vi "Add Element.vi"(8 "Error In":errorcluster, 10 "New Element":refnum<class "Display Element.lvclass">, 11 "Display Manager In":refnum<class "Display Manager.lvclass">) -> (0 "Error Out":errorcluster, 3 "Display Manager Out":refnum<class "Display Manager.lvclass">)   [LabVIEW 2021, in "Display Manager.lvclass"]
uses:
  Display Manager.lvclass
  Display Element/Display Element.lvclass
  Accessors/Display Elements/Get Display Elements.vi
  Accessors/Display Elements/Set Display Elements.vi
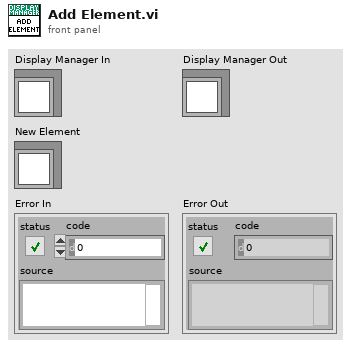
[diagram p1: front panel]
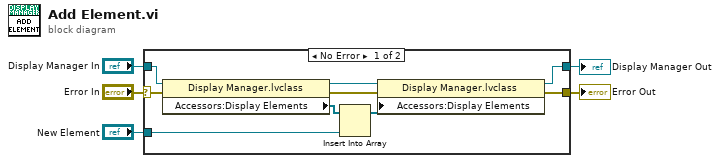
[diagram p0: block diagram]
diagram:
  n1 = case shown="No Error" "Error In" {
    selector: "Error In" -> [w13 w15]
    tunnel: "Display Manager In" -> [w14 w16]
    tunnel: [w10 w16] -> w3
    tunnel: [w11 w15] -> w2
    tunnel: "New Element" -> [w7 _]
    frame No Error {
      n2 = property class="Display Manager.lvclass"(reference=w14, error in=w13) -> (reference out=w12:refnum<class "Display Manager.lvclass">, error out=w8:errorcluster, "Accessors:Display Elements"=w9:refnum<class "Display Element.lvclass">[])
      n3 = Insert Into Array(array=w9, new element=w7) -> (w6:refnum<class "Display Element.lvclass">[])  [unwired: 1 in]
      n4 = property class="Display Manager.lvclass"(reference=w12, error in=w8, "Accessors:Display Elements"=w6) -> (reference out=w10:refnum<class "Display Manager.lvclass">, error out=w11:errorcluster)
    }
    frame Error {
    }
  }
  "Display Manager Out" <- w3
  "Error Out" <- w2
